vi "LED Loop.vi"   [LabVIEW 2017]
uses:
  Common Code/Intake States.ctl
  Robot Global Data.vi
types:
  T1 = typedef "Intake States.ctl" = enum16{"Curl Up", "Override Angle", "Idle", "Drop Mid", "Drop Low", "Outtake", "Intake"}
  T2 = typedef "Drivetrain Status Cluster.ctl" = cluster{"Throttle (Y)":dbl, "Steer (X)":dbl, "Drivetrain Mode":T3, "Brake?":bool, "Distance Drive Complete?":bool, "PID Drive Complete?":bool, "Creep Mode?":bool, "Gyro Steer Complete?":bool, "Gyro":dbl, "X Max Output":dbl, "X Min Output":dbl, "Y Max Output ":dbl, "Y Min Output":dbl, "Heading Target":dbl, "Distance Target":dbl, "Gear 2":bool, "Drivetrain Encoder Values":T4}
  T3 = typedef "Drivetrain Mode.ctl" = enum16{"Manual", "Gyro Steer", "PID Drive", "Distance Drive", "Autonomous"}
  T4 = typedef "DT Encoder Values.ctl" = cluster{"Left Encoder":cluster{"Distance":dbl, "Speed":dbl, "Tick":dbl}, "Right Encoder":cluster{"Distance":dbl, "Speed":dbl, "Tick":dbl}}
  T5 = typedef "Intake Status Cluster.ctl" = cluster{"Intake Mode":T6, "Intake States":T1, "Intake Current Angle":dbl, "Cube In Posession?":bool}
  T6 = typedef "Intake Mode.ctl" = enum16{"Auto", "Semi Auto", "Manual"}
  T7 = typedef "Elevator Status Cluster.ctl" = cluster{"Finished":bool, "Output":dbl, "Elevator State":T8, "Elevator Mode":T9, "Encoder Height":dbl, "Elevator Height":dbl, "At Bottom?":bool, "At Top?":bool}
  T8 = typedef "Elevator State.ctl" = enum16{"Idle", "Ground", "Mid", "Scale", "Switch"}
  T9 = typedef "Elevator Mode.ctl" = enum16{"Semi Auto", "Manual", "Auto"}
  T10 = typedef "WPI_DriverStationRobotMode2.ctl" = enum16{"Autonomous Disabled", "Autonomous Enabled", "Teleop Disabled", "Teleop Enabled", "Disconnected", "Finish", "Test Disabled", "Test Enabled", "Emergency Stopped"}
  T11 = typedef "WPI_I2CDevRef.ctl" = cluster{"DevStatus":errorcluster, "Device Address":u8, "Handle":i32, "I2C Bus":T12}
  T12 = typedef "i2c_bus.ctl" = enum16{"I2C On-Board", "I2C MXP", "Invalid"}
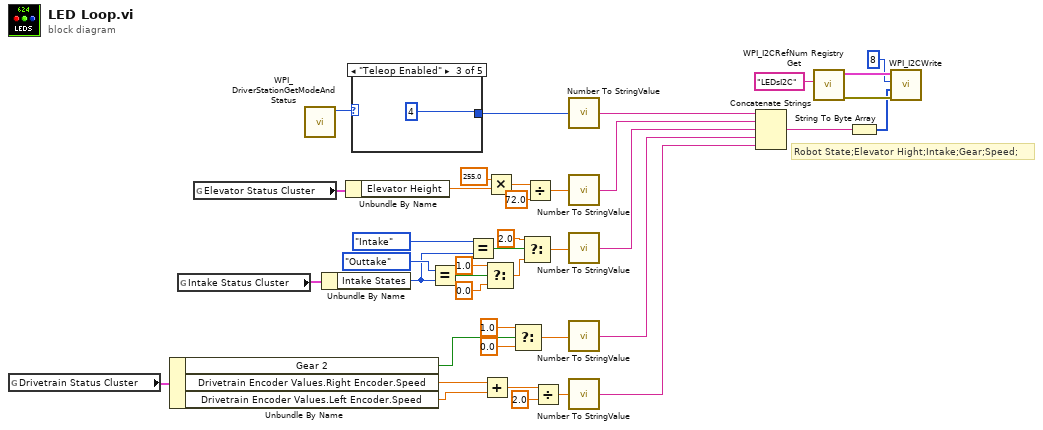
[diagram p0: block diagram]
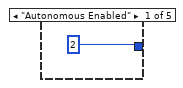
[diagram p2: hidden frame]
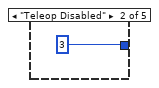
[diagram p3: hidden frame]
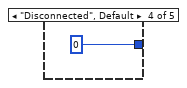
[diagram p4: hidden frame]
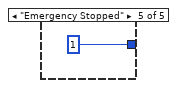
[diagram p5: hidden frame]
diagram:
  # "Robot State;Elevator Hight;Intake;Gear;Speed;"
  n1 = global read "Robot Global Data.vi" "Drivetrain Status Cluster"() -> (w12:T2)
  n2 = Unbundle By Name(w12) -> ("Gear 2"=w11:bool, "Drivetrain Encoder Values.Right Encoder.Speed"=w6:dbl, "Drivetrain Encoder Values.Left Encoder.Speed"=w5:dbl)
  n3 = global read "Robot Global Data.vi" "Intake Status Cluster"() -> (w30:T5)
  n4 = global read "Robot Global Data.vi" "Elevator Status Cluster"() -> (w31:T7)
  n5 = call <vilib>:"WPI_DriverStationGetModeAndStatus.vi"() -> ("Robot Mode"=w40:T10)  [unwired: 10 in, 1 out]
  n6 = Unbundle By Name(w30) -> ("Intake States"=w24:T1)
  n7 = Unbundle By Name(w31) -> ("Elevator Height"=w18:dbl)
  n8 = case shown="\"Teleop Enabled\"" w40 {
    tunnel: [2 3 4 0 1] -> w34
    frame "Autonomous Enabled" {
    }
    frame "Teleop Disabled" {
    }
    frame "Teleop Enabled" {
    }
    frame "Disconnected", Default {
    }
    frame "Emergency Stopped" {
    }
  }
  n9 = Equal?(x=Intake_States."Outtake" ("Intake States"), y=w24) -> (x = y?=w28:bool)
  n10 = Equal?(x=Intake_States."Intake" ("Intake States"), y=w24) -> (x = y?=w27:bool)
  n11 = Add(x=w6, y=w5) -> (x+y=w4:dbl)
  n12 = Select(t=1.0, s=w28, f=0.0) -> (s? t:f=w29:dbl)
  n13 = Multiply(x=255.0, y=w18) -> (x*y=w17:dbl)
  n14 = Select(t=1.0, s=w11, f=0.0) -> (s? t:f=w8:dbl)
  n15 = Select(t=2.0, s=w27, f=w29) -> (s? t:f=w20:dbl)
  n16 = Divide(x=w17, y=72.0) -> (x/y=w14:dbl)
  n17 = Divide(x=w4, y=2.0) -> (x/y=w2:dbl)
  n18 = call "Number To StringValue.vi"("Number In"=w34) -> ("String Out"=w32:string)
  n19 = call "Number To StringValue.vi"("Number In"=w14) -> ("String Out"=w13:string)
  n20 = call "Number To StringValue.vi"("Number In"=w20) -> ("String Out"=w19:string)
  n21 = call "Number To StringValue.vi"("Number In"=w8) -> ("String Out"=w7:string)
  n22 = call "Number To StringValue.vi"("Number In"=w2) -> ("String Out"=w1:string)
  n23 = Concatenate Strings(w32, w13, w19, w7, w1) -> (w33:string)
  n24 = call <vilib>:"WPI_I2CRefNum Registry Get.vi"("refnum name"="LEDsI2C") -> ("error out"=w37:errorcluster, "I2CDevRef"=w38:T11)  [unwired: 9 in]
  n25 = String To Byte Array(string=w33) -> (unsigned byte array=w35:u8[])
  n26 = call <vilib>:"WPI_I2CWrite.vi"("error in (no error)"=w37, "I2CDataToSend"=w35, "I2CRegister"=u8 8, "I2CDevRef"=w38) -> ()  [unwired: 6 in, 2 out]
